vi "Lab Panel V4.89.vi"() -> ()   [LabVIEW 2013] (continued)
                                n569 = Build Array("Testers Name", "Description", "Set Test Cycles", "T-Rise minutes", "T-Rise Deg C") -> (w892:string[])
                                n570 = Unbundle(w891) -> ("NAME"=w890:string, "DESCRIPTION"=w889:string, "CYCLES"=w888:dbl, "T-RISE mins"=w887:dbl, "T-RISE deg C"=w886:dbl)
                                n571 = Number To Decimal String(number=w888) -> (decimal integer string=w901:string)  [unwired: 1 in]
                                n572 = Number To Decimal String(number=w887) -> (decimal integer string=w900:string)  [unwired: 1 in]
                                n573 = Number To Decimal String(number=w886) -> (decimal integer string=w899:string)  [unwired: 1 in]
                                n574 = Build Array(w890, w889, w901, w900, w899) -> (w898:string[])
                                n575 = TDMS Set Properties(5:w898, 7:w892, 11:w902) -> ()  [unwired: 3 in, 4 out]
                              }
                              frame #3 {
                                n576 = local read "DISP LAB01-2"() -> (w904:T4)
                                n577 = Concatenate Strings("LAB01-2  ", w907) -> (w908:string)
                                n578 = Two Button Dialog(message=w908, 1:w905, 2:w906) -> (T button?=w910:bool)
                                n579 = case shown="True" w910 {
                                tunnel: w904 -> [w917 w918]
                                tunnel: [w917 w918] -> w914
                                tunnel: [w916 w919] -> w913
                                tunnel: [w915 w919] -> w912
                                frame False {
                                n580 = Unbundle(w917) -> ("CYCLE"=w916:dbl, "MINS"=w915:dbl)  [unwired: 1 out]
                                }
                                frame True {
                                w919 = 0.0
                                }
                                }
                                n581 = Bundle(cluster=w914, "CYCLE"=w913, "MINS"=w912, "STATUS"="RUN") -> (w903:T4)
                                n582 = local write "DISP LAB01-2"(w903) -> ()
                              }
                              frame #4 {
                                n583 = local read "TEMP START LAB01-2"() -> (w922:cluster{"TL":dbl, "TN":dbl})
                                n584 = Bundle(cluster=w922, "TL"=w920, "TN"=w920) -> (w921:cluster{"TL":dbl, "TN":dbl})
                                n585 = local write "TEMP START LAB01-2"(w921) -> ()
                              }
                            }
                          }
                        }
                      }
                    }
                  }
                }
              }
              event "RUN LAB02-1": Value Change {
                n586 = event-data() -> ("NewVal"=w928:bool)  [unwired: 1 in, 5 out]
                n587 = local read "SIG LAB02-1"() -> (w924:T2)
                n588 = case shown="True" w928 {
                  tunnel: w934 -> [_ w972]
                  tunnel: w933 -> [_ w971]
                  tunnel: w931 -> [w936 w970]
                  tunnel: w932 -> [_ w969]
                  tunnel: w930 -> [_ w968]
                  tunnel: [w935 w967] -> w929
                  tunnel: w927 -> [_ w966]
                  tunnel: w926 -> [_ w965]
                  tunnel: w925 -> [_ w964]
                  tunnel: w924 -> [_ w963]
                  tunnel: w923 -> [_ w962]
                  frame False {
                    # "stop test"
                    n589 = stacked-sequence {
                      tunnel: w936 -> [w945 _]
                      tunnel: [w937 _] -> w935
                      frame #0 {
                        n590 = local read "DISP LAB02-1"() -> (w944:T4)
                        n591 = Unbundle(w944) -> ("CYCLE"=w942:dbl, "MINS"=w943:dbl)  [unwired: 1 out]
                        n592 = case shown="\"CYCLE TEST\"" w945 {
                          tunnel: w943 -> [_ _ w952]
                          tunnel: w942 -> [w950 w951 _]
                          tunnel: [w950 w951 w952] -> w941
                          frame "CHART TEST", Default {
                          }
                          frame "CYCLE TEST" {
                          }
                          frame "T-RISE TEST" {
                          }
                        }
                        n593 = local read "TDMS LAB02-1"() -> (w949:refnum<k34>)
                        n594 = Build Array("STOPPED") -> (w946:string[])
                        n595 = Build Array(w941) -> (w940:dbl[])
                        n596 = TDMS Write(0:w949, 5:"TEST RESULT", 7:w946, 9:w940) -> (4:w938:refnum<k34>, 15:w939:errorcluster)  [unwired: 2 in, 2 out]
                        n597 = TDMS Close(8:w939, 11:w938) -> (0:w937:errorcluster)  [unwired: 1 out]
                      }
                      frame #1 {
                        n598 = local read "DISP LAB02-1"() -> (w956:T4)
                        n599 = stacked-sequence {
                          tunnel: "LAB02-1" -> [w958 w960]
                          frame #0 {
                            n600 = call "sub vi - defrag tdms v1.vi"("panel id"=w958) -> ("error out"=w957:errorcluster)  [unwired: 10 in]
                            n601 = local write "data file error"(w957) -> ()
                          }
                          frame #1 {
                            n602 = local write "RESULT LAB02-1"(FALSE) -> ()
                            n603 = call "Save data file (stop) v3.vi"("panel id"=w960) -> ("network file save error"=w959:errorcluster)  [unwired: 9 in, 1 out]
                            n604 = local write "data file error"(w959) -> ()
                          }
                        }
                        n605 = Bundle(cluster=w956, "STATUS"="STOP") -> (w954:T4)  [unwired: 2 in]
                        n606 = local write "DISP LAB02-1"(w954) -> ()
                      }
                    }
                  }
                  frame True {
                    n607 = stacked-sequence {
                      seq-local: [w974 _] -> [_ w978]
                      tunnel: w972 -> [_ w988]
                      tunnel: w971 -> [_ w987]
                      tunnel: w970 -> [_ w986]
                      tunnel: w969 -> [_ w985]
                      tunnel: w968 -> [_ w984]
                      tunnel: [_ w983] -> w967
                      tunnel: w966 -> [_ w982]
                      tunnel: w965 -> [_ w981]
                      tunnel: w964 -> [_ w980]
                      tunnel: w963 -> [w973 w979]
                      tunnel: w962 -> [_ w977]
                      frame #0 {
                        n608 = Unbundle(w973) -> ("AMPS"=w976:dbl)  [unwired: 4 out]
                        n609 = call "Check For Amps on v1.vi"("ID"="LAB02-1", "amps"=w976) -> ("amps"=w974:bool)  [unwired: 9 in]
                      }
                      frame #1 {
                        n610 = case shown="True" w978 {
                          tunnel: w988 -> [_ w1001]
                          tunnel: w987 -> [_ w1000]
                          tunnel: w986 -> [_ w999]
                          tunnel: w985 -> [_ w998]
                          tunnel: w984 -> [_ w997]
                          tunnel: [errorcluster {"status"=FALSE, "code"=0, "source"=""} ("error out") w996] -> w983
                          tunnel: w982 -> [_ w995]
                          tunnel: w981 -> [_ w994]
                          tunnel: w980 -> [_ w993]
                          tunnel: w979 -> [_ w992]
                          tunnel: w977 -> [_ w991]
                          frame False {
                            w990 = FALSE
                            n611 = local write "RUN LAB02-1"(w990) -> ()
                            n612 = local write "run lab02-1"(w990) -> ()
                          }
                          frame True {
                            n613 = stacked-sequence {
                              seq-local: [w1002 _ _ _ _] -> [_ w1026 _ _ _]
                              tunnel: w1001 -> [w1007 _ _ _ _]
                              tunnel: w1000 -> [w1004 _ _ _ _]
                              tunnel: w999 -> [w1017 _ _ _ _]
                              tunnel: w998 -> [w1010 _ _ _ _]
                              tunnel: w997 -> [w1005 _ _ _ _]
                              tunnel: [_ w1021 _ _ _] -> w996
                              tunnel: w995 -> [_ _ _ w1047 _]
                              tunnel: w994 -> [_ _ _ w1046 _]
                              tunnel: w993 -> [_ _ _ w1045 _]
                              tunnel: w992 -> [_ _ _ _ _]
                              tunnel: w991 -> [_ _ _ _ w1061]
                              frame #0 {
                                w1003 = "\\"
                                n614 = local read "SET LAB02-1"() -> (w1012:T5)
                                n615 = case shown="\"CYCLE TEST\"" w1017 {
                                tunnel: ["L02-1-CHART TEST-" "L02-1-CYCLE TEST-" "L02-1-T-RISE TEST-"] -> w1013
                                frame "CHART TEST", Default {
                                }
                                frame "CYCLE TEST" {
                                }
                                frame "T-RISE TEST" {
                                }
                                }
                                n616 = Unbundle(w1012) -> ("DESCRIPTION"=w1011:string)  [unwired: 4 out]
                                n617 = Concatenate Strings(w1007, "\\", w1005, w1003, w1004, w1003) -> (w1014:string)
                                n618 = String To Path(string=w1014) -> (path=w1016:path)
                                n619 = Concatenate Strings(w1014, w1013, w1011, "-", w1010, ".tdms") -> (w1002:string)
                                n620 = Create Folder(path (use dialog)=w1016) -> (error out=w1015:errorcluster)  [unwired: 2 in, 2 out]
                                n621 = global write "Global 1.vi" "LAB02-1 FILE"(w1002) -> ()
                                n622 = call <vilib>:"Clear Errors.vi"("error in (no error)"=w1015) -> ()  [unwired: 6 in, 1 out]
                              }
                              frame #1 {
                                (unwired) FALSE
                                n623 = String To Path(string=w1026) -> (path=w1022:path)
                                n624 = TDMS Open(6:FALSE, 10:T20."create or replace" ("operation (0:open)"), 11:w1022) -> (0:w1021:errorcluster, 3:→"TDMS LAB02-1":refnum<k34>)  [unwired: 4 in]
                              }
                              frame #2 {
                                n625 = local read "SET LAB02-1"() -> (w1032:T5)
                                n626 = local read "TDMS LAB02-1"() -> (w1043:refnum<k34>)
                                n627 = Build Array("Testers Name", "Description", "Set Test Cycles", "T-Rise minutes", "T-Rise Deg C") -> (w1033:string[])
                                n628 = Unbundle(w1032) -> ("NAME"=w1031:string, "DESCRIPTION"=w1030:string, "CYCLES"=w1029:dbl, "T-RISE mins"=w1028:dbl, "T-RISE deg C"=w1027:dbl)
                                n629 = Number To Decimal String(number=w1029) -> (decimal integer string=w1042:string)  [unwired: 1 in]
                                n630 = Number To Decimal String(number=w1028) -> (decimal integer string=w1041:string)  [unwired: 1 in]
                                n631 = Number To Decimal String(number=w1027) -> (decimal integer string=w1040:string)  [unwired: 1 in]
                                n632 = Build Array(w1031, w1030, w1042, w1041, w1040) -> (w1039:string[])
                                n633 = TDMS Set Properties(5:w1039, 7:w1033, 11:w1043) -> ()  [unwired: 3 in, 4 out]
                              }
                              frame #3 {
                                n634 = local read "DISP LAB02-1"() -> (w1048:T4)
                                n635 = Concatenate Strings("LAB02-1  ", w1047) -> (w1049:string)
                                n636 = Two Button Dialog(message=w1049, 1:w1045, 2:w1046) -> (T button?=w1051:bool)
                                n637 = case shown="True" w1051 {
                                tunnel: w1048 -> [w1058 w1059]
                                tunnel: [w1058 w1059] -> w1055
                                tunnel: [w1057 w1060] -> w1054
                                tunnel: [w1056 w1060] -> w1053
                                frame False {
                                n638 = Unbundle(w1058) -> ("CYCLE"=w1057:dbl, "MINS"=w1056:dbl)  [unwired: 1 out]
                                }
                                frame True {
                                w1060 = 0.0
                                }
                                }
                                n639 = Bundle(cluster=w1055, "CYCLE"=w1054, "MINS"=w1053, "STATUS"="RUN") -> (w1044:T4)
                                n640 = local write "DISP LAB02-1"(w1044) -> ()
                              }
                              frame #4 {
                                n641 = local read "TEMP START LAB02-1"() -> (w1063:cluster{"TL":dbl, "TN":dbl})
                                n642 = Bundle(cluster=w1063, "TL"=w1061, "TN"=w1061) -> (w1062:cluster{"TL":dbl, "TN":dbl})
                                n643 = local write "TEMP START LAB02-1"(w1062) -> ()
                              }
                            }
                          }
                        }
                      }
                    }
                  }
                }
                n644 = local write "run lab02-1"(w928) -> ()
              }
              event "RUN LAB02-2": Value Change {
                n645 = event-data() -> ("NewVal"=w1068:bool)  [unwired: 1 in, 5 out]
                n646 = local write "run lab02-2"(w1068) -> ()
                n647 = case shown="True" w1068 {
                  tunnel: w1074 -> [_ w1112]
                  tunnel: w1073 -> [_ w1111]
                  tunnel: w1071 -> [w1076 w1110]
                  tunnel: w1072 -> [_ w1109]
                  tunnel: w1070 -> [_ w1108]
                  tunnel: [w1075 w1107] -> w1069
                  tunnel: w1067 -> [_ w1106]
                  tunnel: w1066 -> [_ w1105]
                  tunnel: w1065 -> [_ w1104]
                  tunnel: w1064 -> [_ w1102]
                  frame False {
                    # "stop test"
                    n648 = stacked-sequence {
                      tunnel: w1076 -> [w1085 _]
                      tunnel: [w1077 _] -> w1075
                      frame #0 {
                        n649 = local read "DISP LAB02-2"() -> (w1084:T4)
                        n650 = Unbundle(w1084) -> ("CYCLE"=w1082:dbl, "MINS"=w1083:dbl)  [unwired: 1 out]
                        n651 = case shown="\"CYCLE TEST\"" w1085 {
                          tunnel: w1083 -> [_ _ w1092]
                          tunnel: w1082 -> [w1090 w1091 _]
                          tunnel: [w1090 w1091 w1092] -> w1081
                          frame "CHART TEST", Default {
                          }
                          frame "CYCLE TEST" {
                          }
                          frame "T-RISE TEST" {
                          }
                        }
                        n652 = local read "TDMS LAB02-2"() -> (w1089:refnum<k34>)
                        n653 = Build Array("STOPPED") -> (w1086:string[])
                        n654 = Build Array(w1081) -> (w1080:dbl[])
                        n655 = TDMS Write(0:w1089, 5:"TEST RESULT", 7:w1086, 9:w1080) -> (4:w1078:refnum<k34>, 15:w1079:errorcluster)  [unwired: 2 in, 2 out]
                        n656 = TDMS Close(8:w1079, 11:w1078) -> (0:w1077:errorcluster)  [unwired: 1 out]
                      }
                      frame #1 {
                        n657 = local read "DISP LAB02-2"() -> (w1096:T4)
                        n658 = stacked-sequence {
                          tunnel: "LAB02-2" -> [w1098 w1100]
                          frame #0 {
                            n659 = call "sub vi - defrag tdms v1.vi"("panel id"=w1098) -> ("error out"=w1097:errorcluster)  [unwired: 10 in]
                            n660 = local write "data file error"(w1097) -> ()
                          }
                          frame #1 {
                            n661 = call "Save data file (stop) v3.vi"("panel id"=w1100) -> ("network file save error"=w1099:errorcluster)  [unwired: 9 in, 1 out]
                            n662 = local write "RESULT LAB02-2"(FALSE) -> ()
                            n663 = local write "data file error"(w1099) -> ()
                          }
                        }
                        n664 = Bundle(cluster=w1096, "STATUS"="STOP") -> (w1094:T4)  [unwired: 2 in]
                        n665 = local write "DISP LAB02-2"(w1094) -> ()
                      }
                    }
                  }
                  frame True {
                    n666 = local read "SIG LAB02-2"() -> (w1103:T2)
                    n667 = stacked-sequence {
                      seq-local: [w1114 _] -> [_ w1118]
                      tunnel: w1112 -> [_ w1128]
                      tunnel: w1111 -> [_ w1127]
                      tunnel: w1110 -> [_ w1126]
                      tunnel: w1109 -> [_ w1125]
                      tunnel: w1108 -> [_ w1124]
                      tunnel: [_ w1123] -> w1107
                      tunnel: w1106 -> [_ w1122]
                      tunnel: w1105 -> [_ w1121]
                      tunnel: w1104 -> [_ w1120]
                      tunnel: w1103 -> [w1113 w1119]
                      tunnel: w1102 -> [_ w1117]
                      frame #0 {
                        n668 = Unbundle(w1113) -> ("AMPS"=w1116:dbl)  [unwired: 4 out]
                        n669 = call "Check For Amps on v1.vi"("ID"="LAB02-2", "amps"=w1116) -> ("amps"=w1114:bool)  [unwired: 9 in]
                      }
                      frame #1 {
                        n670 = case shown="True" w1118 {
                          tunnel: w1128 -> [_ w1141]
                          tunnel: w1127 -> [_ w1140]
                          tunnel: w1126 -> [_ w1139]
                          tunnel: w1125 -> [_ w1138]
                          tunnel: w1124 -> [_ w1137]
                          tunnel: [errorcluster {"status"=FALSE, "code"=0, "source"=""} ("error out") w1136] -> w1123
                          tunnel: w1122 -> [_ w1135]
                          tunnel: w1121 -> [_ w1134]
                          tunnel: w1120 -> [_ w1133]
                          tunnel: w1119 -> [_ w1132]
                          tunnel: w1117 -> [_ w1131]
                          frame False {
                            w1129 = FALSE
                            n671 = local write "RUN LAB02-2"(w1129) -> ()
                            n672 = local write "run lab02-2"(w1129) -> ()
                          }
                          frame True {
                            n673 = stacked-sequence {
                              seq-local: [w1142 _ _ _ _] -> [_ w1166 _ _ _]
                              tunnel: w1141 -> [w1147 _ _ _ _]
                              tunnel: w1140 -> [w1144 _ _ _ _]
                              tunnel: w1139 -> [w1157 _ _ _ _]
                              tunnel: w1138 -> [w1150 _ _ _ _]
                              tunnel: w1137 -> [w1145 _ _ _ _]
                              tunnel: [_ w1161 _ _ _] -> w1136
                              tunnel: w1135 -> [_ _ _ w1187 _]
                              tunnel: w1134 -> [_ _ _ w1186 _]
                              tunnel: w1133 -> [_ _ _ w1185 _]
                              tunnel: w1132 -> [_ _ _ _ _]
                              tunnel: w1131 -> [_ _ _ _ w1201]
                              frame #0 {
                                w1143 = "\\"
                                n674 = local read "SET LAB02-2"() -> (w1152:T5)
                                n675 = case shown="\"CYCLE TEST\"" w1157 {
                                tunnel: ["L02-2-CHART TEST-" "L02-2-CYCLE TEST-" "L02-2-T-RISE TEST-"] -> w1153
                                frame "CHART TEST", Default {
                                }
                                frame "CYCLE TEST" {
                                }
                                frame "T-RISE TEST" {
                                }
                                }
                                n676 = Unbundle(w1152) -> ("DESCRIPTION"=w1151:string)  [unwired: 4 out]
                                n677 = Concatenate Strings(w1147, "\\", w1145, w1143, w1144, w1143) -> (w1154:string)
                                n678 = String To Path(string=w1154) -> (path=w1156:path)
                                n679 = Concatenate Strings(w1154, w1153, w1151, "-", w1150, ".tdms") -> (w1142:string)
                                n680 = Create Folder(path (use dialog)=w1156) -> (error out=w1155:errorcluster)  [unwired: 2 in, 2 out]
                                n681 = global write "Global 1.vi" "LAB02-2 FILE"(w1142) -> ()
                                n682 = call <vilib>:"Clear Errors.vi"("error in (no error)"=w1155) -> ()  [unwired: 6 in, 1 out]
                              }
                              frame #1 {
                                (unwired) FALSE
                                n683 = String To Path(string=w1166) -> (path=w1162:path)
                                n684 = TDMS Open(6:FALSE, 10:T20."create or replace" ("operation (0:open)"), 11:w1162) -> (0:w1161:errorcluster, 3:→"TDMS LAB02-2":refnum<k34>)  [unwired: 4 in]
                              }
                              frame #2 {
                                n685 = local read "SET LAB02-2"() -> (w1172:T5)
                                n686 = local read "TDMS LAB02-2"() -> (w1183:refnum<k34>)
                                n687 = Build Array("Testers Name", "Description", "Set Test Cycles", "T-Rise minutes", "T-Rise Deg C") -> (w1173:string[])
                                n688 = Unbundle(w1172) -> ("NAME"=w1171:string, "DESCRIPTION"=w1170:string, "CYCLES"=w1169:dbl, "T-RISE mins"=w1168:dbl, "T-RISE deg C"=w1167:dbl)
                                n689 = Number To Decimal String(number=w1169) -> (decimal integer string=w1182:string)  [unwired: 1 in]
                                n690 = Number To Decimal String(number=w1168) -> (decimal integer string=w1181:string)  [unwired: 1 in]
                                n691 = Number To Decimal String(number=w1167) -> (decimal integer string=w1180:string)  [unwired: 1 in]
                                n692 = Build Array(w1171, w1170, w1182, w1181, w1180) -> (w1179:string[])
                                n693 = TDMS Set Properties(5:w1179, 7:w1173, 11:w1183) -> ()  [unwired: 3 in, 4 out]
                              }
                              frame #3 {
                                n694 = local read "DISP LAB02-2"() -> (w1188:T4)
                                n695 = Concatenate Strings("LAB02-2  ", w1187) -> (w1189:string)
                                n696 = Two Button Dialog(message=w1189, 1:w1185, 2:w1186) -> (T button?=w1191:bool)
                                n697 = case shown="True" w1191 {
                                tunnel: w1188 -> [w1198 w1199]
                                tunnel: [w1198 w1199] -> w1195
                                tunnel: [w1197 w1200] -> w1194
                                tunnel: [w1196 w1200] -> w1193
                                frame False {
                                n698 = Unbundle(w1198) -> ("CYCLE"=w1197:dbl, "MINS"=w1196:dbl)  [unwired: 1 out]
                                }
                                frame True {
                                w1200 = 0.0
                                }
                                }
                                n699 = Bundle(cluster=w1195, "CYCLE"=w1194, "MINS"=w1193, "STATUS"="RUN") -> (w1184:T4)
                                n700 = local write "DISP LAB02-2"(w1184) -> ()
                              }
                              frame #4 {
                                n701 = local read "TEMP START LAB02-2"() -> (w1203:cluster{"TL":dbl, "TN":dbl})
                                n702 = Bundle(cluster=w1203, "TL"=w1201, "TN"=w1201) -> (w1202:cluster{"TL":dbl, "TN":dbl})
                                n703 = local write "TEMP START LAB02-2"(w1202) -> ()
                              }
                            }
                          }
                        }
                      }
                    }
                  }
                }
              }
              event "RUN LAB03-1": Value Change {
                n704 = event-data() -> ("NewVal"=w1208:bool)  [unwired: 1 in, 5 out]
                n705 = local write "run lab03-1"(w1208) -> ()
                n706 = case shown="True" w1208 {
                  tunnel: w1214 -> [_ w1252]
                  tunnel: w1213 -> [_ w1251]
                  tunnel: w1211 -> [w1216 w1250]
                  tunnel: w1212 -> [_ w1249]
                  tunnel: w1210 -> [_ w1248]
                  tunnel: [w1215 w1247] -> w1209
                  tunnel: w1207 -> [_ w1246]
                  tunnel: w1206 -> [_ w1245]
                  tunnel: w1205 -> [_ w1244]
                  tunnel: w1204 -> [_ w1242]
                  frame False {
                    # "stop test"
                    n707 = stacked-sequence {
                      tunnel: w1216 -> [w1225 _]
                      tunnel: [w1217 _] -> w1215
                      frame #0 {
                        n708 = local read "DISP LAB03-1"() -> (w1224:T4)
                        n709 = Unbundle(w1224) -> ("CYCLE"=w1222:dbl, "MINS"=w1223:dbl)  [unwired: 1 out]
                        n710 = case shown="\"CYCLE TEST\"" w1225 {
                          tunnel: w1223 -> [_ _ w1232]
                          tunnel: w1222 -> [w1230 w1231 _]
                          tunnel: [w1230 w1231 w1232] -> w1221
                          frame "CHART TEST", Default {
                          }
                          frame "CYCLE TEST" {
                          }
                          frame "T-RISE TEST" {
                          }
                        }
                        n711 = local read "TDMS LAB03-1"() -> (w1229:refnum<k34>)
                        n712 = Build Array("STOPPED") -> (w1226:string[])
                        n713 = Build Array(w1221) -> (w1220:dbl[])
                        n714 = TDMS Write(0:w1229, 5:"TEST RESULT", 7:w1226, 9:w1220) -> (4:w1218:refnum<k34>, 15:w1219:errorcluster)  [unwired: 2 in, 2 out]
                        n715 = TDMS Close(8:w1219, 11:w1218) -> (0:w1217:errorcluster)  [unwired: 1 out]
                      }
                      frame #1 {
                        n716 = local read "DISP LAB03-1"() -> (w1236:T4)
                        n717 = stacked-sequence {
                          tunnel: "LAB03-1" -> [w1238 w1240]
                          frame #0 {
                            n718 = call "sub vi - defrag tdms v1.vi"("panel id"=w1238) -> ("error out"=w1237:errorcluster)  [unwired: 10 in]
                            n719 = local write "data file error"(w1237) -> ()
                          }
                          frame #1 {
                            n720 = call "Save data file (stop) v3.vi"("panel id"=w1240) -> ("network file save error"=w1239:errorcluster)  [unwired: 9 in, 1 out]
                            n721 = local write "RESULT LAB03-1"(FALSE) -> ()
                            n722 = local write "data file error"(w1239) -> ()
                          }
                        }
                        n723 = Bundle(cluster=w1236, "STATUS"="STOP") -> (w1234:T4)  [unwired: 2 in]
                        n724 = local write "DISP LAB03-1"(w1234) -> ()
                      }
                    }
                  }
                  frame True {
                    n725 = local read "SIG LAB03-1"() -> (w1243:T2)
                    n726 = stacked-sequence {
                      seq-local: [w1254 _] -> [_ w1258]
                      tunnel: w1252 -> [_ w1268]
                      tunnel: w1251 -> [_ w1267]
                      tunnel: w1250 -> [_ w1266]
                      tunnel: w1249 -> [_ w1265]
                      tunnel: w1248 -> [_ w1264]
                      tunnel: [_ w1263] -> w1247
                      tunnel: w1246 -> [_ w1262]
                      tunnel: w1245 -> [_ w1261]
                      tunnel: w1244 -> [_ w1260]
                      tunnel: w1243 -> [w1253 w1259]
                      tunnel: w1242 -> [_ w1257]
                      frame #0 {
                        n727 = Unbundle(w1253) -> ("AMPS"=w1256:dbl)  [unwired: 4 out]
                        n728 = call "Check For Amps on v1.vi"("ID"="LAB03-1", "amps"=w1256) -> ("amps"=w1254:bool)  [unwired: 9 in]
                      }
                      frame #1 {
                        n729 = case shown="True" w1258 {
                          tunnel: w1268 -> [_ w1281]
                          tunnel: w1267 -> [_ w1280]
                          tunnel: w1266 -> [_ w1279]
                          tunnel: w1265 -> [_ w1278]
                          tunnel: w1264 -> [_ w1277]
                          tunnel: [errorcluster {"status"=FALSE, "code"=0, "source"=""} ("error out") w1276] -> w1263
                          tunnel: w1262 -> [_ w1275]
                          tunnel: w1261 -> [_ w1274]
                          tunnel: w1260 -> [_ w1273]
                          tunnel: w1259 -> [_ w1272]
                          tunnel: w1257 -> [_ w1271]
                          frame False {
                            w1269 = FALSE
                            n730 = local write "RUN LAB03-1"(w1269) -> ()
                            n731 = local write "run lab03-1"(w1269) -> ()
                          }
                          frame True {
                            n732 = stacked-sequence {
                              seq-local: [w1282 _ _ _ _] -> [_ w1306 _ _ _]
                              tunnel: w1281 -> [w1287 _ _ _ _]
                              tunnel: w1280 -> [w1284 _ _ _ _]
                              tunnel: w1279 -> [w1297 _ _ _ _]
                              tunnel: w1278 -> [w1290 _ _ _ _]
                              tunnel: w1277 -> [w1285 _ _ _ _]
                              tunnel: [_ w1301 _ _ _] -> w1276
                              tunnel: w1275 -> [_ _ _ w1326 _]
                              tunnel: w1274 -> [_ _ _ w1325 _]
                              tunnel: w1273 -> [_ _ _ w1324 _]
                              tunnel: w1272 -> [_ _ _ _ _]
                              tunnel: w1271 -> [_ _ _ _ w1341]
                              frame #0 {
                                w1283 = "\\"
                                n733 = local read "SET LAB03-1"() -> (w1292:T5)
                                n734 = case shown="\"T-RISE TEST\"" w1297 {
                                tunnel: ["L03-1-CHART TEST-" "L03-1-CYCLE TEST-" "L03-1-T-RISE TEST-"] -> w1293
                                frame "CHART TEST", Default {
                                }
                                frame "CYCLE TEST" {
                                }
                                frame "T-RISE TEST" {
                                }
                                }
                                n735 = Unbundle(w1292) -> ("DESCRIPTION"=w1291:string)  [unwired: 4 out]
                                n736 = Concatenate Strings(w1287, "\\", w1285, w1283, w1284, w1283) -> (w1294:string)
                                n737 = String To Path(string=w1294) -> (path=w1296:path)
                                n738 = Concatenate Strings(w1294, w1293, w1291, "-", w1290, ".tdms") -> (w1282:string)
                                n739 = Create Folder(path (use dialog)=w1296) -> (error out=w1295:errorcluster)  [unwired: 2 in, 2 out]
                                n740 = global write "Global 1.vi" "LAB03-1 FILE"(w1282) -> ()
                                n741 = call <vilib>:"Clear Errors.vi"("error in (no error)"=w1295) -> ()  [unwired: 6 in, 1 out]
                              }
                              frame #1 {
                                (unwired) FALSE
                                n742 = String To Path(string=w1306) -> (path=w1302:path)
                                n743 = TDMS Open(6:FALSE, 10:T20."create or replace" ("operation (0:open)"), 11:w1302) -> (0:w1301:errorcluster, 3:→"TDMS LAB03-1":refnum<k34>)  [unwired: 4 in]
                              }
                              frame #2 {
                                n744 = local read "SET LAB03-1"() -> (w1312:T5)
                                n745 = local read "TDMS LAB03-1"() -> (w1323:refnum<k34>)
                                n746 = Build Array("Testers Name", "Description", "Set Test Cycles", "T-Rise minutes", "T-Rise Deg C") -> (w1313:string[])
                                n747 = Unbundle(w1312) -> ("NAME"=w1311:string, "DESCRIPTION"=w1310:string, "CYCLES"=w1309:dbl, "T-RISE mins"=w1308:dbl, "T-RISE deg C"=w1307:dbl)
                                n748 = Number To Decimal String(number=w1309) -> (decimal integer string=w1322:string)  [unwired: 1 in]
                                n749 = Number To Decimal String(number=w1308) -> (decimal integer string=w1321:string)  [unwired: 1 in]
                                n750 = Number To Decimal String(number=w1307) -> (decimal integer string=w1320:string)  [unwired: 1 in]
                                n751 = Build Array(w1311, w1310, w1322, w1321, w1320) -> (w1319:string[])
                                n752 = TDMS Set Properties(5:w1319, 7:w1313, 11:w1323) -> ()  [unwired: 3 in, 4 out]
                              }
                              frame #3 {
                                n753 = local read "DISP LAB03-1"() -> (w1328:T4)
                                n754 = Concatenate Strings("LAB03-1  ", w1326) -> (w1329:string)
                                n755 = Two Button Dialog(message=w1329, 1:w1324, 2:w1325) -> (T button?=w1331:bool)
                                n756 = case shown="True" w1331 {
                                tunnel: w1328 -> [w1338 w1339]
                                tunnel: [w1338 w1339] -> w1335
                                tunnel: [w1337 w1340] -> w1334
                                tunnel: [w1336 w1340] -> w1333
                                frame False {
                                n757 = Unbundle(w1338) -> ("CYCLE"=w1337:dbl, "MINS"=w1336:dbl)  [unwired: 1 out]
                                }
                                frame True {
                                w1340 = 0.0
                                }
                                }
                                n758 = Bundle(cluster=w1335, "CYCLE"=w1334, "MINS"=w1333, "STATUS"="RUN") -> (w1327:T4)
                                n759 = local write "DISP LAB03-1"(w1327) -> ()
                              }
                              frame #4 {
                                n760 = local read "TEMP START LAB03-1"() -> (w1343:cluster{"TL":dbl, "TN":dbl})
                                n761 = Bundle(cluster=w1343, "TL"=w1341, "TN"=w1341) -> (w1342:cluster{"TL":dbl, "TN":dbl})
                                n762 = local write "TEMP START LAB03-1"(w1342) -> ()
                              }
                            }
                          }
                        }
                      }
                    }
                  }
                }
              }
              event "RUN LAB03-2": Value Change {
                n763 = event-data() -> ("NewVal"=w1348:bool)  [unwired: 1 in, 5 out]
                n764 = local write "run lab03-2"(w1348) -> ()
                n765 = case shown="True" w1348 {
                  tunnel: w1354 -> [_ w1392]
                  tunnel: w1353 -> [_ w1391]
                  tunnel: w1351 -> [w1356 w1390]
                  tunnel: w1352 -> [_ w1389]
                  tunnel: w1350 -> [_ w1388]
                  tunnel: [w1355 w1387] -> w1349
                  tunnel: w1347 -> [_ w1386]
                  tunnel: w1346 -> [_ w1385]
                  tunnel: w1345 -> [_ w1384]
                  tunnel: w1344 -> [_ w1382]
                  frame False {
                    # "stop test"
                    n766 = stacked-sequence {
                      tunnel: w1356 -> [w1365 _]
                      tunnel: [w1357 _] -> w1355
                      frame #0 {
                        n767 = local read "DISP LAB03-2"() -> (w1364:T4)
                        n768 = Unbundle(w1364) -> ("CYCLE"=w1362:dbl, "MINS"=w1363:dbl)  [unwired: 1 out]
                        n769 = case shown="\"CYCLE TEST\"" w1365 {
                          tunnel: w1363 -> [_ _ w1372]
                          tunnel: w1362 -> [w1370 w1371 _]
                          tunnel: [w1370 w1371 w1372] -> w1361
                          frame "CHART TEST", Default {
                          }
                          frame "CYCLE TEST" {
                          }
                          frame "T-RISE TEST" {
                          }
                        }
                        n770 = local read "TDMS LAB03-2"() -> (w1369:refnum<k34>)
                        n771 = Build Array("STOPPED") -> (w1366:string[])
                        n772 = Build Array(w1361) -> (w1360:dbl[])
                        n773 = TDMS Write(0:w1369, 5:"TEST RESULT", 7:w1366, 9:w1360) -> (4:w1358:refnum<k34>, 15:w1359:errorcluster)  [unwired: 2 in, 2 out]
                        n774 = TDMS Close(8:w1359, 11:w1358) -> (0:w1357:errorcluster)  [unwired: 1 out]
                      }
                      frame #1 {
                        n775 = local read "DISP LAB03-2"() -> (w1376:T4)
                        n776 = stacked-sequence {
                          tunnel: "LAB03-2" -> [w1378 w1380]
                          frame #0 {
                            n777 = call "sub vi - defrag tdms v1.vi"("panel id"=w1378) -> ("error out"=w1377:errorcluster)  [unwired: 10 in]
                            n778 = local write "data file error"(w1377) -> ()
                          }
                          frame #1 {
                            n779 = call "Save data file (stop) v3.vi"("panel id"=w1380) -> ("network file save error"=w1379:errorcluster)  [unwired: 9 in, 1 out]
                            n780 = local write "RESULT LAB03-2"(FALSE) -> ()
                            n781 = local write "data file error"(w1379) -> ()
                          }
                        }
                        n782 = Bundle(cluster=w1376, "STATUS"="STOP") -> (w1374:T4)  [unwired: 2 in]
                        n783 = local write "DISP LAB03-2"(w1374) -> ()
                      }
                    }
                  }
                  frame True {
                    n784 = local read "SIG LAB03-2"() -> (w1383:T2)
                    n785 = stacked-sequence {
                      seq-local: [w1394 _] -> [_ w1398]
                      tunnel: w1392 -> [_ w1408]
                      tunnel: w1391 -> [_ w1407]
                      tunnel: w1390 -> [_ w1406]
                      tunnel: w1389 -> [_ w1405]
                      tunnel: w1388 -> [_ w1404]
                      tunnel: [_ w1403] -> w1387
                      tunnel: w1386 -> [_ w1402]
                      tunnel: w1385 -> [_ w1401]
                      tunnel: w1384 -> [_ w1400]
                      tunnel: w1383 -> [w1393 w1399]
                      tunnel: w1382 -> [_ w1397]
                      frame #0 {
                        n786 = Unbundle(w1393) -> ("AMPS"=w1396:dbl)  [unwired: 4 out]
                        n787 = call "Check For Amps on v1.vi"("ID"="LAB03-2", "amps"=w1396) -> ("amps"=w1394:bool)  [unwired: 9 in]
                      }
                      frame #1 {
                        n788 = case shown="True" w1398 {
                          tunnel: w1408 -> [_ w1421]
                          tunnel: w1407 -> [_ w1420]
                          tunnel: w1406 -> [_ w1419]
                          tunnel: w1405 -> [_ w1418]
                          tunnel: w1404 -> [_ w1417]
                          tunnel: [errorcluster {"status"=FALSE, "code"=0, "source"=""} ("error out") w1416] -> w1403
                          tunnel: w1402 -> [_ w1415]
                          tunnel: w1401 -> [_ w1414]
                          tunnel: w1400 -> [_ w1413]
                          tunnel: w1399 -> [_ w1412]
                          tunnel: w1397 -> [_ w1411]
                          frame False {
                            w1409 = FALSE
                            n789 = local write "RUN LAB03-2"(w1409) -> ()
                            n790 = local write "run lab03-2"(w1409) -> ()
                          }
                          frame True {
                            n791 = stacked-sequence {
                              seq-local: [w1422 _ _ _ _] -> [_ w1446 _ _ _]
                              tunnel: w1421 -> [w1427 _ _ _ _]
                              tunnel: w1420 -> [w1424 _ _ _ _]
                              tunnel: w1419 -> [w1437 _ _ _ _]
                              tunnel: w1418 -> [w1430 _ _ _ _]
                              tunnel: w1417 -> [w1425 _ _ _ _]
                              tunnel: [_ w1441 _ _ _] -> w1416
                              tunnel: w1415 -> [_ _ _ w1467 _]
                              tunnel: w1414 -> [_ _ _ w1466 _]
                              tunnel: w1413 -> [_ _ _ w1465 _]
                              tunnel: w1412 -> [_ _ _ _ _]
                              tunnel: w1411 -> [_ _ _ _ w1481]
                              frame #0 {
                                w1423 = "\\"
                                n792 = local read "SET LAB03-2"() -> (w1432:T5)
                                n793 = case shown="\"T-RISE TEST\"" w1437 {
                                tunnel: ["L03-2-CHART TEST-" "L03-2-CYCLE TEST-" "L03-2-T-RISE TEST-"] -> w1433
                                frame "CHART TEST", Default {
                                }
                                frame "CYCLE TEST" {
                                }
                                frame "T-RISE TEST" {
                                }
                                }
                                n794 = Unbundle(w1432) -> ("DESCRIPTION"=w1431:string)  [unwired: 4 out]
                                n795 = Concatenate Strings(w1427, "\\", w1425, w1423, w1424, w1423) -> (w1434:string)
                                n796 = String To Path(string=w1434) -> (path=w1436:path)
                                n797 = Concatenate Strings(w1434, w1433, w1431, "-", w1430, ".tdms") -> (w1422:string)
                                n798 = Create Folder(path (use dialog)=w1436) -> (error out=w1435:errorcluster)  [unwired: 2 in, 2 out]
                                n799 = global write "Global 1.vi" "LAB03-2 FILE"(w1422) -> ()
                                n800 = call <vilib>:"Clear Errors.vi"("error in (no error)"=w1435) -> ()  [unwired: 6 in, 1 out]
                              }
                              frame #1 {
                                (unwired) FALSE
                                n801 = String To Path(string=w1446) -> (path=w1442:path)
                                n802 = TDMS Open(6:FALSE, 10:T20."create or replace" ("operation (0:open)"), 11:w1442) -> (0:w1441:errorcluster, 3:→"TDMS LAB03-2":refnum<k34>)  [unwired: 4 in]
                              }
                              frame #2 {
                                n803 = local read "SET LAB03-2"() -> (w1452:T5)
                                n804 = local read "TDMS LAB03-2"() -> (w1463:refnum<k34>)
                                n805 = Build Array("Testers Name", "Description", "Set Test Cycles", "T-Rise minutes", "T-Rise Deg C") -> (w1453:string[])
                                n806 = Unbundle(w1452) -> ("NAME"=w1451:string, "DESCRIPTION"=w1450:string, "CYCLES"=w1449:dbl, "T-RISE mins"=w1448:dbl, "T-RISE deg C"=w1447:dbl)
                                n807 = Number To Decimal String(number=w1449) -> (decimal integer string=w1462:string)  [unwired: 1 in]
                                n808 = Number To Decimal String(number=w1448) -> (decimal integer string=w1461:string)  [unwired: 1 in]
                                n809 = Number To Decimal String(number=w1447) -> (decimal integer string=w1460:string)  [unwired: 1 in]
                                n810 = Build Array(w1451, w1450, w1462, w1461, w1460) -> (w1459:string[])
                                n811 = TDMS Set Properties(5:w1459, 7:w1453, 11:w1463) -> ()  [unwired: 3 in, 4 out]
                              }
                              frame #3 {
                                n812 = local read "DISP LAB03-2"() -> (w1468:T4)
                                n813 = Concatenate Strings("LAB03-2  ", w1467) -> (w1469:string)
                                n814 = Two Button Dialog(message=w1469, 1:w1465, 2:w1466) -> (T button?=w1471:bool)
                                n815 = case shown="True" w1471 {
                                tunnel: w1468 -> [w1478 w1479]
                                tunnel: [w1478 w1479] -> w1475
                                tunnel: [w1477 w1480] -> w1474
                                tunnel: [w1476 w1480] -> w1473
                                frame False {
                                n816 = Unbundle(w1478) -> ("CYCLE"=w1477:dbl, "MINS"=w1476:dbl)  [unwired: 1 out]
                                }
                                frame True {
                                w1480 = 0.0
                                }
                                }
                                n817 = Bundle(cluster=w1475, "CYCLE"=w1474, "MINS"=w1473, "STATUS"="RUN") -> (w1464:T4)
                                n818 = local write "DISP LAB03-2"(w1464) -> ()
                              }
                              frame #4 {
                                n819 = local read "TEMP START LAB03-2"() -> (w1483:cluster{"TL":dbl, "TN":dbl})
                                n820 = Bundle(cluster=w1483, "TL"=w1481, "TN"=w1481) -> (w1482:cluster{"TL":dbl, "TN":dbl})
                                n821 = local write "TEMP START LAB03-2"(w1482) -> ()
                              }
                            }
                          }
                        }
                      }
                    }
                  }
                }
              }
              event "RUN LAB04-1": Value Change {
                n822 = event-data() -> ("NewVal"=w1488:bool)  [unwired: 1 in, 5 out]
                n823 = local write "run lab04-1"(w1488) -> ()
                n824 = case shown="True" w1488 {
                  tunnel: w1494 -> [_ w1532]
                  tunnel: w1493 -> [_ w1531]
                  tunnel: w1491 -> [w1496 w1530]
                  tunnel: w1492 -> [_ w1529]
                  tunnel: w1490 -> [_ w1528]
                  tunnel: [w1495 w1527] -> w1489
                  tunnel: w1487 -> [_ w1526]
                  tunnel: w1486 -> [_ w1525]
                  tunnel: w1485 -> [_ w1524]
                  tunnel: w1484 -> [_ w1522]
                  frame False {
                    # "stop test"
                    n825 = stacked-sequence {
                      tunnel: w1496 -> [w1505 _]
                      tunnel: [w1497 _] -> w1495
                      frame #0 {
                        n826 = local read "DISP LAB04-1"() -> (w1504:T4)
                        n827 = Unbundle(w1504) -> ("CYCLE"=w1502:dbl, "MINS"=w1503:dbl)  [unwired: 1 out]
                        n828 = case shown="\"CYCLE TEST\"" w1505 {
                          tunnel: w1503 -> [_ _ w1512]
                          tunnel: w1502 -> [w1510 w1511 _]
                          tunnel: [w1510 w1511 w1512] -> w1501
                          frame "CHART TEST", Default {
                          }
                          frame "CYCLE TEST" {
                          }
                          frame "T-RISE TEST" {
                          }
                        }
                        n829 = local read "TDMS LAB04-1"() -> (w1509:refnum<k34>)
                        n830 = Build Array("STOPPED") -> (w1506:string[])
                        n831 = Build Array(w1501) -> (w1500:dbl[])
                        n832 = TDMS Write(0:w1509, 5:"TEST RESULT", 7:w1506, 9:w1500) -> (4:w1498:refnum<k34>, 15:w1499:errorcluster)  [unwired: 2 in, 2 out]
                        n833 = TDMS Close(8:w1499, 11:w1498) -> (0:w1497:errorcluster)  [unwired: 1 out]
                      }
                      frame #1 {
                        n834 = local read "DISP LAB04-1"() -> (w1516:T4)
                        n835 = stacked-sequence {
                          tunnel: "LAB04-1" -> [w1518 w1520]
                          frame #0 {
                            n836 = call "sub vi - defrag tdms v1.vi"("panel id"=w1518) -> ("error out"=w1517:errorcluster)  [unwired: 10 in]
                            n837 = local write "data file error"(w1517) -> ()
                          }
                          frame #1 {
                            n838 = call "Save data file (stop) v3.vi"("panel id"=w1520) -> ("network file save error"=w1519:errorcluster)  [unwired: 9 in, 1 out]
                            n839 = local write "RESULT LAB04-1"(FALSE) -> ()
                            n840 = local write "data file error"(w1519) -> ()
                          }
                        }
                        n841 = Bundle(cluster=w1516, "STATUS"="STOP") -> (w1514:T4)  [unwired: 2 in]
                        n842 = local write "DISP LAB04-1"(w1514) -> ()
                      }
                    }
                  }
                  frame True {
                    n843 = local read "SIG LAB04-1"() -> (w1523:T2)
